vi "log analysis_gps.vi"() -> ()   [LabVIEW 2018] (continued)
,0.0976,0.1029,4.9518,0f000001,0*3a7eab6c\n\tsystem status\tnormal 2 27.800000 0 0\trobot status\t227.318577\t105.493966\t8.215100\t0.358371\t-1.600174\t171.393514\t0.252000\t0.087000\n\t\n15:37:15.7\tlog_raw\tgps_raw\t#INSPVAXA,USB3,0,48.5,FINESTEERING,2107,283053.700,02000000,471d,15824;INS_ALIGNMENT_COMPLETE,INS_RTKFIXED,37.37108102802,126.72339980538,8.2112,22.3000,0.0729,-0.2744,-0.0174,0.330552076,-1.494765101,278.139995916,0.4480,0.2956,0.5639,0.1143,0.0926,0.0779,0.0976,0.1029,4.9518,0f000001,0*6b892211\n\tsystem status\tnormal 2 27.800000 0 0\trobot status\t227.176950\t105.524570\t8.211200\t0.330552\t-1.494765\t171.860004\t0.412000\t-0.165000\n\t\n15:37:16.2\tlog_raw\tgps_raw\t#DUALANTENNAHEADINGA,USB3,0,45.5,FINESTEERING,2107,283054.200,02000000,d426,15824;INSUFFICIENT_OBS,NONE,-1.000000000,0.000000000,0.000000000,0.0,0.000000000,0.000000000,\"631T\",19,2,2,2,04,00,20,00*86f4b129\n\tsystem status\tnormal 2 27.800000 0 0\trobot status\t227.035841\t105.555084\t8.206800\t0.430368\t-1.501164\t172.299734\t0.195000\t0.158000\n\t\n15:37:16.7\tlog_raw\tgps_raw\t#INSPVAXA,USB3,0,45.5,FINESTEERING,2107,283054.700,02000000,471d,15824;INS_ALIGNMENT_COMPLETE,INS_RTKFIXED,37.37108154829,126.72339665209,8.2035,22.3000,0.0578,-0.2607,-0.0176,0.280593250,-1.428439620,277.446082188,0.4484,0.2957,0.5646,0.1144,0.0926,0.0779,0.0976,0.1029,4.9527,0f000001,0*8d0f64c8\n\tsystem status\tnormal 2 27.900000 0 0\trobot status\t226.897637\t105.582319\t8.203500\t0.280593\t-1.428440\t172.553918\t0.233000\t0.103000\n\t\n15:37:17.2\tlog_raw\tgps_raw\t#INSPVAXA,USB3,0,46.0,FINESTEERING,2107,283055.200,02000000,471d,15824;INS_ALIGNMENT_COMPLETE,INS_RTKFIXED,37.37108179458,126.72339508506,8.2008,22.3000,0.0590,-0.2687,-0.0093,0.251526173,-1.446507840,277.289322874,0.4481,0.2956,0.5644,0.1143,0.0926,0.0779,0.0976,0.1029,4.9538,0f000001,0*05040f15\n\tsystem status\tnormal 2 27.900000 0 0\trobot status\t226.758832\t105.609657\t8.200800\t0.251526\t-1.446508\t172.710677\t0.330000\t-0.056000\n\t\n15:37:17.7\tlog_raw\tgps_raw\t#INSPVAXA,USB3,0,46.0,FINESTEERING,2107,283055.700,02000000,471d,15824;INS_ALIGNMENT_COMPLETE,INS_RTKFIXED,37.37108204101,126.72339350294,8.1980,22.3000,0.0573,-0.2710,-0.0141,0.338881932,-1.408720439,277.315135363,0.4481,0.2956,0.5644,0.1143,0.0926,0.0779,0.0976,0.1029,4.9538,0f000001,0*6debbe04\n\tsystem status\tnormal 2 27.900000 0 0\trobot status\t226.618691\t105.637011\t8.198000\t0.338882\t-1.408720\t172.684865\t0.289000\t0.007000\n\t\n15:37:18.2\tlog_raw\tgps_raw\t#INSPVAXA,USB3,0,52.0,FINESTEERING,2107,283056.200,02000000,471d,15824;INS_ALIGNMENT_COMPLETE,INS_RTKFIXED,37.37108228588,126.72339196103,8.1952,22.3000,0.0487,-0.2508,-0.0076,0.405017158,-1.170976426,277.337977168,0.4477,0.2956,0.5639,0.1144,0.0926,0.0778,0.0976,0.1028,4.9548,0f000001,0*8b541580\n\tsystem status\tnormal 2 27.900000 0 0\trobot status\t226.482111\t105.664192\t8.195200\t0.405017\t-1.170976\t172.662023\t0.253000\t0.037000\n\t\n15:37:18.7\tlog_raw\tgps_raw\t#DUALANTENNAHEADINGA,USB3,0,52.0,FINESTEERING,2107,283056.700,02000000,d426,15824;INSUFFICIENT_OBS,NONE,-1.000000000,0.000000000,0.000000000,0.0,0.000000000,0.000000000,\"631T\",13,2,2,2,04,00,20,00*95485060\n\tsystem status\tnormal 2 28.000000 0 0\trobot status\t226.354812\t105.690997\t8.192600\t0.493668\t-1.115925\t172.765731\t0.208000\t0.011000\n\t\n15:37:19.2\tlog_raw\tgps_raw\t#DUALANTENNAHEADINGA,USB3,0,50.0,FINESTEERING,2107,283057.200,02000000,d426,15824;INSUFFICIENT_OBS,NONE,-1.000000000,0.000000000,0.000000000,0.0,0.000000000,0.000000000,\"631T\",13,2,2,2,04,00,20,00*e70ae8a8\n\tsystem status\tnormal 2 27.900000 0 0\trobot status\t226.254411\t105.711039\t8.190300\t0.338108\t-0.961096\t172.566593\t0.336000\t0.019000\n\t\n15:37:19.7\tlog_raw\tgps_raw\t#DUALANTENNAHEADINGA,USB3,0,50.0,FINESTEERING,2107,283057.700,02000000,d426,15824;INSUFFICIENT_OBS,NONE,-1.000000000,0.000000000,0.000000000,0.0,0.000000000,0.000000000,\"631T\",13,2,2,2,04,00,20,00*3019f9f1\n\tsystem status\tnormal 2 28.000000 0 0\trobot status\t226.091572\t105.739836\t8.186700\t0.308993\t-0.921996\t172.531902\t0.231000\t-0.008000\n\t\n15:37:20.2\tlog_raw\tgps_raw\t#INSPVAXA,USB3,0,52.0,FINESTEERING,2107,283058.200,02000000,471d,15824;INS_ALIGNMENT_COMPLETE,INS_RTKFIXED,37.37108315467,126.72338641713,8.1848,22.3000,0.0560,-0.2718,-0.0107,0.129590736,-0.819774204,277.698102716,0.4474,0.2955,0.5631,0.1155,0.0927,0.0778,0.0975,0.1028,4.9554,0f000001,0*a6d9a945\n\tsystem status\tnormal 2 27.900000 0 0\trobot status\t225.991041\t105.760627\t8.184800\t0.129591\t-0.819774\t172.301897\t0.296000\t-0.040000\n\t\n15:37:20.7\tlog_raw\tgps_raw\t#INSPVAXA,USB3,0,52.0,FINESTEERING,2107,283058.700,02000000,471d,15824;INS_ALIGNMENT_COMPLETE,INS_RTKFIXED,37.37108344441,126.72338455262,8.1832,22.3000,0.0621,-0.2653,-0.0184,0.032268015,-0.987434909,277.857905932,0.4474,0.2955,0.5631,0.1155,0.0927,0.0778,0.0975,0.1028,4.9554,0f000001,0*0fff6d0e\n\tsystem status\tnormal 2 28.000000 0 0\trobot status\t225.825886\t105.792788\t8.183200\t0.032268\t-0.987435\t172.142094\t0.338000\t0.019000\n\t\n15:37:21.2\tlog_raw\tgps_raw\t#INSPVAXA,USB3,0,51.0,FINESTEERING,2107,283059.200,02000000,471d,15824;INS_ALIGNMENT_COMPLETE,INS_RTKFIXED,37.37108373104,126.72338298116,8.1814,22.3000,0.0640,-0.2840,-0.0248,0.084962299,-0.861930897,278.528163453,0.4480,0.2954,0.5625,0.1142,0.0926,0.0777,0.0975,0.1027,4.9533,0f000001,0*55180826\n\tsystem status\tnormal 2 27.900000 0 0\trobot status\t225.686688\t105.824604\t8.181400\t0.084962\t-0.861931\t171.471837\t0.294000\t-0.065000\n\t\n15:37:21.7\tlog_raw\tgps_raw\t#INSPVAXA,USB3,0,51.0,FINESTEERING,2107,283059.700,02000000,471d,15824;INS_ALIGNMENT_COMPLETE,INS_RTKFIXED,37.37108405973,126.72338145683,8.1789,22.3000,0.0766,-0.2838,-0.0077,0.302314246,-0.745003967,279.694826311,0.4480,0.2954,0.5625,0.1142,0.0926,0.0777,0.0975,0.1027,4.9533,0f000001,0*c3a85521\n\tsystem status\tnormal 2 27.800000 0 0\trobot status\t225.551666\t105.861087\t8.178900\t0.302314\t-0.745004\t170.305174\t0.268000\t-0.122000\n\t\n15:37:22.2\tlog_raw\tgps_raw\t#DUALANTENNAHEADINGA,USB3,0,49.5,FINESTEERING,2107,283060.200,02000000,d426,15824;INSUFFICIENT_OBS,NONE,-1.000000000,0.000000000,0.000000000,0.0,0.000000000,0.000000000,\"631T\",14,2,2,2,04,00,20,00*d9be019d\n\tsystem status\tnormal 2 27.700000 0 0\trobot status\t225.411173\t105.899741\t8.176500\t0.188888\t-0.758738\t168.859131\t0.270000\t-0.100000\n\t\n15:37:22.7\tlog_raw\tgps_raw\t#INSPVAXA,USB3,0,49.5,FINESTEERING,2107,283060.700,02000000,471d,15824;INS_ALIGNMENT_COMPLETE,INS_RTKFIXED,37.37108477080,126.72337829109,8.1755,22.3000,0.0829,-0.2746,-0.0191,-0.114275154,-0.865621982,282.712324181,0.4478,0.2952,0.5620,0.1144,0.0926,0.0777,0.0975,0.1027,4.9522,0f000001,0*f5ce6e6a\n\tsystem status\tnormal 2 27.700000 0 0\trobot status\t225.271250\t105.940012\t8.175500\t-0.114275\t-0.865622\t167.287676\t0.300000\t-0.060000\n\t\n15:37:23.2\tlog_raw\tgps_raw\t#DUALANTENNAHEADINGA,USB3,0,49.0,FINESTEERING,2107,283061.200,02008000,d426,15824;SOL_COMPUTED,L1_FLOAT,-1.000000000,252.567794800,53.338584900,0.0,294.937744141,135.460769653,\"631T\",15,6,6,6,04,00,20,23*fbe42f58\n\tsystem status\tnormal 2 27.600000 0 0\trobot status\t225.132703\t105.985425\t8.176200\t-0.269945\t-1.010706\t165.810739\t0.300000\t-0.051000\n\t\n15:37:23.7\tlog_raw\tgps_raw\t#DUALANTENNAHEADINGA,USB3,0,49.0,FINESTEERING,2107,283061.700,02008000,d426,15824;INSUFFICIENT_OBS,NONE,-1.000000000,0.000000000,0.000000000,0.0,0.000000000,0.000000000,\"631T\",13,2,2,2,04,00,20,00*6aa2fd3b\n\tsystem status\tnormal 2 27.700000 0 0\trobot status\t224.997401\t106.035994\t8.177700\t-0.281716\t-0.789311\t164.588174\t0.297000\t-0.033000\n\t\n15:37:24.2\tlog_raw\tgps_raw\t#DUALANTENNAHEADINGA,USB3,0,45.5,FINESTEERING,2107,283062.200,02008000,d426,15824;INSUFFICIENT_OBS,NONE,-1.000000000,0.000000000,0.000000000,0.0,0.000000000,0.000000000,\"631T\",13,2,2,2,04,00,20,00*8005e2b6\n\tsystem status\tnormal 2 27.700000 0 0\trobot status\t224.859892\t106.090568\t8.178500\t-0.217716\t-0.817210\t163.548657\t0.247000\t-0.094000\n\t\n15:37:24.7\tlog_raw\tgps_raw\t#DUALANTENNAHEADINGA,USB3,0,45.5,FINESTEERING,2107,283062.700,02008000,d426,15824;INSUFFICIENT_OBS,NONE,-1.000000000,0.000000000,0.000000000,0.0,0.000000000,0.000000000,\"631T\",13,2,2,2,04,00,20,00*5716f3ef\n\tsystem status\tnormal 2 27.800000 0 0\trobot status\t224.725412\t106.145668\t8.178100\t-0.361245\t-0.626933\t162.778759\t0.341000\t0.060000\n\t\n15:37:25.2\tlog_raw\tgps_raw\t#DUALANTENNAHEADINGA,USB3,0,46.0,FINESTEERING,2107,283063.200,02008000,d426,15824;INSUFFICIENT_OBS,NONE,-1.000000000,0.000000000,0.000000000,0.0,0.000000000,0.000000000,\"631T\",12,2,2,2,04,00,20,00*c388fb17\n\tsystem status\tnormal 2 27.800000 0 0\trobot status\t224.590934\t106.202616\t8.177500\t-0.366610\t-0.485076\t162.261228\t0.254000\t-0.071000\n\t\n15:37:25.7\tlog_raw\tgps_raw\t#INSPVAXA,USB3,0,46.0,FINESTEERING,2107,283063.700,02008000,471d,15824;INS_ALIGNMENT_COMPLETE,INS_RTKFIXED,37.37108763910,126.72336915850,8.1772,22.3000,0.0613,-0.1484,-0.0057,-0.315544156,-0.705788351,288.188502375,0.4460,0.2952,0.5608,0.1140,0.0926,0.0776,0.0975,0.1026,4.9515,0f000001,0*11521a0a\n\tsystem status\tnormal 2 27.900000 0 0\trobot status\t224.462300\t106.258371\t8.177200\t-0.315544\t-0.705788\t161.811498\t0.183000\t-0.002000\n\t\n15:37:26.2\tlog_raw\tgps_raw\t#DUALANTENNAHEADINGA,USB3,0,49.5,FINESTEERING,2107,283064.200,02008000,d426,15824;INSUFFICIENT_OBS,NONE,-1.000000000,0.000000000,0.000000000,0.0,0.000000000,0.000000000,\"631T\",14,2,2,2,04,00,20,00*a33c9019\n\tsystem status\tnormal 2 28.000000 0 0\trobot status\t224.458512\t106.272057\t8.177700\t-0.418271\t-0.580192\t162.096787\t0.000000\t0.000000\n\t\n15:37:26.7\tlog_raw\tgps_raw\t#DUALANTENNAHEADINGA,USB3,0,49.5,FINESTEERING,2107,283064.700,02008000,d426,15824;INSUFFICIENT_OBS,NONE,-1.000000000,0.000000000,0.000000000,0.0,0.000000000,0.000000000,\"631T\",13,2,2,2,04,00,20,00*3e110a0b\n\tsystem status\tnormal 2 28.000000 0 0\trobot status\t224.462166\t106.283022\t8.179100\t-0.421246\t-0.578710\t162.036915\t0.000000\t0.000000\n\t\n15:37:27.2\tlog_raw\tgps_raw\t#DUALANTENNAHEADINGA,USB3,0,50.0,FINESTEERING,2107,283065.200,02008000,d426,15824;INSUFFICIENT_OBS,NONE,-1.000000000,0.000000000,0.000000000,0.0,0.000000000,0.000000000,\"631T\",13,2,2,2,04,00,20,00*f0ffb566\n\tsystem status\tnormal 2 28.000000 0 0\trobot status\t224.465375\t106.293143\t8.180100\t-0.419277\t-0.578107\t162.046332\t0.000000\t0.000000\n\t\n15:37:27.7\tlog_raw\tgps_raw\t#DUALANTENNAHEADINGA,USB3,0,50.0,FINESTEERING,2107,283065.700,02008000,d426,15824;INSUFFICIENT_OBS,NONE,-1.000000000,0.000000000,0.000000000,0.0,0.000000000,0.000000000,\"631T\",14,2,2,2,04,00,20,00*6dd22f74\n\tsystem status\tnormal 2 28.000000 0 0\trobot status\t224.467251\t106.301137\t8.180600\t-0.418596\t-0.575436\t162.044524\t0.000000\t0.000000\n\t\n15:37:28.2\tlog_raw\tgps_raw\t#DUALANTENNAHEADINGA,USB3,0,47.5,FINESTEERING,2107,283066.200,02000000,d426,15824;INSUFFICIENT_OBS,NONE,-1.000000000,0.000000000,0.000000000,0.0,0.000000000,0.000000000,\"631T\",15,2,2,2,04,00,20,00*afd2d569\n\tsystem status\tnormal 2 28.000000 0 0\trobot status\t224.469165\t106.307513\t8.181000\t-0.417828\t-0.575071\t162.040318\t0.000000\t0.000000\n\t\n15:37:28.7\tlog_raw\tgps_raw\t#INSPVAXA,USB3,0,47.5,FINESTEERING,2107,283066.700,02000000,471d,15824;INS_ALIGNMENT_COMPLETE,INS_RTKFIXED,37.37108811035,126.72336925303,8.1815,22.3000,0.0201,0.0148,-0.0079,-0.417962669,-0.573305874,287.968672901,0.4491,0.2953,0.5602,0.1160,0.0930,0.0776,0.0974,0.1026,4.9384,0f000001,0*010a2d8b\n\tsystem status\tnormal 2 28.000000 0 0\trobot status\t224.470673\t106.310672\t8.181500\t-0.417963\t-0.573306\t162.031327\t0.000000\t0.000000\n\t\n15:37:29.2\tlog_raw\tgps_raw\t#INSPVAXA,USB3,0,49.5,FINESTEERING,2107,283067.200,02000000,471d,15824;INS_ALIGNMENT_COMPLETE,INS_RTKFIXED,37.37108813168,126.72336927578,8.1822,22.3000,0.0181,0.0163,-0.0073,-0.419452547,-0.574416189,287.977918899,0.4495,0.2954,0.5600,0.1153,0.0929,0.0776,0.0974,0.1026,4.9275,0f000001,0*549c769b\n\tsystem status\tnormal 2 28.000000 0 0\trobot status\t224.472688\t106.313040\t8.182200\t-0.419453\t-0.574416\t162.022081\t0.000000\t0.000000\n\t\n15:37:29.7\tlog_raw\tgps_raw\t#DUALANTENNAHEADINGA,USB3,0,49.5,FINESTEERING,2107,283067.700,02000000,d426,15824;INSUFFICIENT_OBS,NONE,-1.000000000,0.000000000,0.000000000,0.0,0.000000000,0.000000000,\"631T\",12,2,2,2,04,00,20,00*49080399\n\tsystem status\tnormal 2 28.000000 0 0\trobot status\t224.474564\t106.313838\t8.183300\t-0.418041\t-0.575113\t162.011465\t0.000000\t0.000000\n\t\n15:37:30.2\tlog_raw\tgps_raw\t#DUALANTENNAHEADINGA,USB3,0,52.0,FINESTEERING,2107,283068.200,02000000,d426,15824;INSUFFICIENT_OBS,NONE,-1.000000000,0.000000000,0.000000000,0.0,0.000000000,0.000000000,\"631T\",10,2,2,2,04,00,20,00*54582190\n\tsystem status\tnormal 2 28.000000 0 0\trobot status\t224.476732\t106.314053\t8.184200\t-0.416762\t-0.574697\t162.002567\t0.000000\t0.000000\n\t\n15:37:30.7\tlog_raw\tgps_raw\t#DUALANTENNAHEADINGA,USB3,0,52.0,FINESTEERING,2107,283068.700,02000000,d426,15824;INSUFFICIENT_OBS,NONE,-1.000000000,0.000000000,0.000000000,0.0,0.000000000,0.000000000,\"631T\",10,2,2,2,04,00,20,00*834b30c9\n\tsystem status\tnormal 2 28.000000 0 0\trobot status\t224.477944\t106.313408\t8.184900\t-0.414613\t-0.574002\t161.993059\t0.000000\t0.000000\n\t\n15:37:31.2\tlog_raw\tgps_raw\t#DUALANTENNAHEADINGA,USB3,0,51.0,FINESTEERING,2107,283069.200,02000000,d426,15824;INSUFFICIENT_OBS,NONE,-1.000000000,0.000000000,0.000000000,0.0,0.000000000,0.000000000,\"631T\",10,2,2,2,04,00,20,00*954d5ea5\n\tsystem status\tnormal 2 28.000000 0 0\trobot status\t224.478944\t106.312623\t8.185800\t-0.413248\t-0.574345\t161.980835\t0.000000\t0.000000\n\t\n15:37:31.7\tlog_raw\tgps_raw\t#DUALANTENNAHEADINGA,USB3,0,51.0,FINESTEERING,2107,283069.700,02000000,d426,15824;INSUFFICIENT_OBS,NONE,-1.000000000,0.000000000,0.000000000,0.0,0.000000000,0.000000000,\"631T\",10,2,2,2,04,00,20,00*425e4ffc\n\tsystem status\tnormal 2 28.000000 0 0\trobot status\t224.478622\t106.311286\t8.187100\t-0.413743\t-0.575972\t161.971285\t0.000000\t0.000000\n\t\n15:37:32.2\tlog_raw\tgps_raw\t#DUALANTENNAHEADINGA,USB3,0,52.5,FINESTEERING,2107,283070.200,02000000,d426,15824;INSUFFICIENT_OBS,NONE,-1.000000000,0.000000000,0.000000000,0.0,0.000000000,0.000000000,\"631T\",10,2,2,2,04,00,20,00*26625f62\n\tsystem status\tnormal 2 28.000000 0 0\trobot status\t224.472931\t106.304441\t8.191500\t-0.413676\t-0.576142\t161.957409\t0.000000\t0.000000\n\t\n15:37:32.7\tlog_raw\tgps_raw\t#DUALANTENNAHEADINGA,USB3,0,52.5,FINESTEERING,2107,283070.700,02000000,d426,15824;INSUFFICIENT_OBS,NONE,-1.000000000,0.000000000,0.000000000,0.0,0.000000000,0.000000000,\"631T\",13,2,2,2,04,00,20,00*5227c892\n\tsystem status\tnormal 2 28.000000 0 0\trobot status\t224.457049\t106.286388\t8.201500\t-0.415988\t-0.580830\t161.940237\t0.000000\t0.000000\n\t\n15:37:33.2\tlog_raw\tgps_raw\t#DUALANTENNAHEADINGA,USB3,0,54.5,FINESTEERING,2107,283071.200,02000000,d426,15824;INSUFFICIENT_OBS,NONE,-1.000000000,0.000000000,0.000000000,0.0,0.000000000,0.000000000,\"631T\",13,2,2,2,04,00,20,00*6a072c8b\n\tsystem status\tnormal 2 28.000000 0 0\trobot status\t224.446581\t106.274894\t8.208600\t-0.417440\t-0.583830\t161.929639\t0.000000\t0.000000\n\t\n15:37:33.7\tlog_raw\tgps_raw\t\tsystem status\tnormal 2 28.000000 0 0\trobot status\t224.445080\t106.274741\t8.210500\t-0.413663\t-0.584668\t161.932180\t0.000000\t0.000000\n\t\n15:37:34.2\tlog_raw\tgps_raw\t#DUALANTENNAHEADINGA,USB3,0,49.5,FINESTEERING,2107,283072.200,02000000,d426,15824;INSUFFICIENT_OBS,NONE,-1.000000000,0.000000000,0.000000000,0.0,0.000000000,0.000000000,\"631T\",11,2,2,2,04,00,20,00*c3e637e1\n\tsystem status\tnormal 2 28.000000 0 0\trobot status\t224.444030\t106.274625\t8.212100\t-0.413003\t-0.586018\t161.934159\t0.000000\t0.000000\n\t\n15:37:34.7\tlog_raw\tgps_raw\t#DUALANTENNAHEADINGA,USB3,0,49.5,FINESTEERING,2107,283072.700,02000000,d426,15824;INSUFFICIENT_OBS,NONE,-1.000000000,0.000000000,0.000000000,0.0,0.000000000,0.000000000,\"631T\",13,2,2,2,04,00,20,00*60412049\n\tsystem status\tnormal 2 28.000000 0 0\trobot status\t224.443743\t106.274758\t8.213100\t-0.410619\t-0.587707\t161.938405\t0.000000\t0.000000\n\t\n15:37:35.2\tlog_raw\tgps_raw\t#DUALANTENNAHEADINGA,USB3,0,45.5,FINESTEERING,2107,283073.200,02000000,d426,15824;INSUFFICIENT_OBS,NONE,-1.000000000,0.000000000,0.000000000,0.0,0.000000000,0.000000000,\"631T\",13,2,2,2,04,00,20,00*042cd0ba\n\tsystem status\tnormal 2 28.000000 0 0\trobot status\t224.443799\t106.274913\t8.214000\t-0.409148\t-0.588494\t161.942929\t0.000000\t0.000000\n\t\n15:37:35.7\tlog_raw\tgps_raw\t#DUALANTENNAHEADINGA,USB3,0,45.5,FINESTEERING,2107,283073.700,02000000,d426,15824;INSUFFICIENT_OBS,NONE,-1.000000000,0.000000000,0.000000000,0.0,0.000000000,0.000000000,\"631T\",14,2,2,2,04,00,20,00*99014aa8\n\tsystem status\tnormal 2 28.000000 0 0\trobot status\t224.443802\t106.275172\t8.214400\t-0.408380\t-0.588614\t161.947579\t0.000000\t0.000000\n\t\n15:37:36.2\tlog_raw\tgps_raw\t#DUALANTENNAHEADINGA,USB3,0,50.0,FINESTEERING,2107,283074.200,02000000,d426,15824;INSUFFICIENT_OBS,NONE,-1.000000000,0.000000000,0.000000000,0.0,0.000000000,0.000000000,\"631T\",14,2,2,2,04,00,20,00*3ee80c21\n\tsystem status\tnormal 2 28.000000 0 0\trobot status\t224.443955\t106.275672\t8.214800\t-0.408998\t-0.591093\t161.953750\t0.000000\t0.000000\n\t\n15:37:36.7\tlog_raw\tgps_raw\t#DUALANTENNAHEADINGA,USB3,0,50.0,FINESTEERING,2107,283074.700,02000000,d426,15824;INSUFFICIENT_OBS,NONE,-1.000000000,0.000000000,0.000000000,0.0,0.000000000,0.000000000,\"631T\",13,2,2,2,04,00,20,00*a3c59633\n\tsystem status\tnormal 2 28.000000 0 0\trobot status\t224.443819\t106.276172\t8.215000\t-0.407165\t-0.589977\t161.958792\t0.000000\t0.000000\n\t\n15:37:37.2\tlog_raw\tgps_raw\t#DUALANTENNAHEADINGA,USB3,0,48.5,FINESTEERING,2107,283075.200,02000000,d426,15824;INSUFFICIENT_OBS,NONE,-1.000000000,0.000000000,0.000000000,0.0,0.000000000,0.000000000,\"631T\",14,2,2,2,04,00,20,00*435174b1\n\tsystem status\tnormal 2 28.000000 0 0\trobot status\t224.443749\t106.276912\t8.215400\t-0.406197\t-0.590364\t161.964407\t0.000000\t0.000000\n\t\n15:37:37.7\tlog_raw\tgps_raw\t#DUALANTENNAHEADINGA,USB3,0,48.5,FINESTEERING,2107,283075.700,02000000,d426,15824;INSUFFICIENT_OBS,NONE,-1.000000000,0.000000000,0.000000000,0.0,0.000000000,0.000000000,\"631T\",14,2,2,2,04,00,20,00*944265e8\n\tsystem status\tnormal 2 28.000000 0 0\trobot status\t224.444106\t106.277977\t8.215900\t-0.403240\t-0.589075\t161.971979\t0.000000\t0.000000\n\t\n15:37:38.2\tlog_raw\tgps_raw\t#DUALANTENNAHEADINGA,USB3,0,37.5,FINESTEERING,2107,283076.200,02000000,d426,15824;INSUFFICIENT_OBS,NONE,-1.000000000,0.000000000,0.000000000,0.0,0.000000000,0.000000000,\"631T\",12,2,2,2,04,00,20,00*42000f60\n\tsystem status\tnormal 2 28.000000 0 0\trobot status\t224.444412\t106.279441\t8.216500\t-0.402469\t-0.590649\t161.978968\t0.000000\t0.000000\n\t\n15:37:38.7\tlog_raw\tgps_raw\t#DUALANTENNAHEADINGA,USB3,0,37.5,FINESTEERING,2107,283076.700,02000000,d426,15824;INSUFFICIENT_OBS,NONE,-1.000000000,0.000000000,0.000000000,0.0,0.000000000,0.000000000,\"631T\",12,2,2,2,04,00,20,00*95131e39\n\tsystem status\tnormal 2 28.000000 0 0\trobot status\t224.444474\t106.280452\t8.217300\t-0.403001\t-0.589091\t161.987676\t0.000000\t0.000000\n\t\n15:37:39.2\tlog_raw\tgps_raw\t#DUALANTENNAHEADINGA,USB3,0,41.5,FINESTEERING,2107,283077.200,02000000,d426,15824;INSUFFICIENT_OBS,NONE,-1.000000000,0.000000000,0.000000000,0.0,0.000000000,0.000000000,\"631T\",13,2,2,2,04,00,20,00*225f994e\n\tsystem status\tnormal 2 28.000000 0 0\trobot status\t224.444454\t106.281759\t8.217900\t-0.403382\t-0.588903\t161.995009\t0.000000\t0.000000\n\t\n15:37:39.7\tlog_raw\tgps_raw\t#DUALANTENNAHEADINGA,USB3,0,41.5,FINESTEERING,2107,283077.700,02000000,d426,15824;INSUFFICIENT_OBS,NONE,-1.000000000,0.000000000,0.000000000,0.0,0.000000000,0.000000000,\"631T\",14,2,2,2,04,00,20,00*bf72035c\n\tsystem status\tnormal 2 28.000000 0 0\trobot status\t224.444326\t106.282784\t8.218400\t-0.402465\t-0.590017\t162.002959\t0.000000\t0.000000\n\t\n15:37:40.2\tlog_raw\tgps_raw\t\tsystem status\tnormal 2 28.000000 0 0\trobot status\t224.444423\t106.283924\t8.218700\t-0.402799\t-0.591657\t162.009798\t0.000000\t0.000000\n\t\n15:37:40.7\tlog_raw\tgps_raw\t#DUALANTENNAHEADINGA,USB3,0,47.5,FINESTEERING,2107,283078.700,02000000,d426,15824;INSUFFICIENT_OBS,NONE,-1.000000000,0.000000000,0.000000000,0.0,0.000000000,0.000000000,\"631T\",14,2,2,2,04,00,20,00*3fc2c0c1\n\tsystem status\tnormal 2 28.000000 0 0\trobot status\t224.444432\t106.284530\t8.218700\t-0.403496\t-0.590478\t162.017828\t0.000000\t0.000000\n\t\n15:37:41.2\tlog_raw\tgps_raw\t#INSPVAXA,USB3,0,47.0,FINESTEERING,2107,283079.250,02008000,471d,15824;INS_ALIGNMENT_COMPLETE,INS_RTKFIXED,37.37108788068,126.72336895793,8.2189,22.3000,0.0088,0.0013,-0.0012,-0.401485866,-0.591652619,287.973728649,0.2375,0.1652,0.3301,0.0344,0.0343,0.0312,0.0796,0.0806,4.8842,0f000005,0*b7c6e88e\n\tsystem status\tnormal 2 28.000000 0 0\trobot status\t224.444534\t106.285183\t8.218900\t-0.401486\t-0.591653\t162.026271\t0.000000\t0.000000\n\t\n15:37:41.7\tlog_raw\tgps_raw\t\tsystem status\tnormal 2 28.000000 0 0\trobot status\t224.445189\t106.285558\t8.219200\t-0.401801\t-0.589988\t162.030580\t0.000000\t0.000000\n\t\n15:37:42.2\tlog_raw\tgps_raw\t#DUALANTENNAHEADINGA,USB3,0,48.5,FINESTEERING,2107,283080.200,02008000,d426,15824;INSUFFICIENT_OBS,NONE,-1.000000000,0.000000000,0.000000000,0.0,0.000000000,0.000000000,\"631T\",14,2,2,2,04,00,20,00*53647ec7\n\tsystem status\tnormal 2 28.000000 0 0\trobot status\t224.445852\t106.286374\t8.219400\t-0.402906\t-0.589159\t162.034861\t0.000000\t0.000000\n\t\n15:37:42.7\tlog_raw\tgps_raw\t\tsystem status\tnormal 2 28.000000 0 0\trobot status\t224.446285\t106.286761\t8.219700\t-0.403955\t-0.586941\t162.040555\t0.000000\t0.000000\n\t\n15:37:43.2\tlog_raw\tgps_raw\t#DUALANTENNAHEADINGA,USB3,0,49.5,FINESTEERING,2107,283081.200,02008000,d426,15824;INSUFFICIENT_OBS,NONE,-1.000000000,0.000000000,0.000000000,0.0,0.000000000,0.000000000,\"631T\",13,2,2,2,04,00,20,00*10c627f1\n\tsystem status\tnormal 2 28.000000 0 0\trobot status\t224.446560\t106.287440\t8.219900\t-0.405217\t-0.586615\t162.044562\t0.000000\t0.000000\n\t\n15:37:43.7\tlog_raw\tgps_raw\t#DUALANTENNAHEADINGA,USB3,0,49.5,FINESTEERING,2107,283081.700,02008000,d426,15824;INSUFFICIENT_OBS,NONE,-1.000000000,0.000000000,0.000000000,0.0,0.000000000,0.000000000,\"631T\",13,2,2,2,04,00,20,00*c7d536a8\n\tsystem status\tnormal 2 28.000000 0 0\trobot status\t224.446108\t106.287608\t8.220600\t-0.406769\t-0.585328\t162.047588\t0.000000\t0.000000\n\t\n15:37:44.2\tlog_raw\tgps_raw\t#INSPVAXA,USB3,0,48.0,FINESTEERING,2107,283082.250,02008000,471d,15824;INS_ALIGNMENT_COMPLETE,INS_RTKFIXED,37.37108790543,126.72336897434,8.2212,22.3000,0.0087,0.0020,-0.0010,-0.406487889,-0.586741608,287.950772341,0.2277,0.1614,0.3135,0.0344,0.0343,0.0312,0.0796,0.0806,4.8871,0f000005,0*4c1cc0b2\n\tsystem status\tnormal 2 28.000000 0 0\trobot status\t224.445987\t106.287930\t8.221200\t-0.406488\t-0.586742\t162.049228\t0.000000\t0.000000\n\t\n15:37:44.7\tlog_raw\tgps_raw\t#DUALANTENNAHEADINGA,USB3,0,48.0,FINESTEERING,2107,283082.700,02008000,d426,15824;INSUFFICIENT_OBS,NONE,-1.000000000,0.000000000,0.000000000,0.0,0.000000000,0.000000000,\"631T\",13,2,2,2,04,00,20,00*40830bab\n\tsystem status\tnormal 2 28.000000 0 0\trobot status\t224.446132\t106.288223\t8.221600\t-0.406755\t-0.585861\t162.050623\t0.000000\t0.000000\n\t\n15:37:45.2\tlog_raw\tgps_raw\t#DUALANTENNAHEADINGA,USB3,0,51.0,FINESTEERING,2107,283083.200,02008000,d426,15824;INSUFFICIENT_OBS,NONE,-1.000000000,0.000000000,0.000000000,0.0,0.000000000,0.000000000,\"631T\",13,2,2,2,04,00,20,00*db17520a\n\tsystem status\tnormal 2 28.000000 0 0\trobot status\t224.446264\t106.288675\t8.222000\t-0.407177\t-0.586377\t162.052509\t0.000000\t0.000000\n\t\n15:37:45.7\tlog_raw\tgps_raw\t#INSPVAXA,USB3,0,51.0,FINESTEERING,2107,283083.750,02008000,471d,15824;INS_ALIGNMENT_COMPLETE,INS_RTKFIXED,37.37108791341,126.72336897923,8.2220,22.3000,0.0085,0.0022,-0.0015,-0.407747547,-0.586428741,287.947615621,0.2254,0.1606,0.3090,0.0344,0.0343,0.0312,0.0797,0.0806,4.8884,0f000005,0*f8c3e66c\n\tsystem status\tnormal 2 28.000000 0 0\trobot status\t224.446420\t106.288816\t8.222000\t-0.407748\t-0.586429\t162.052384\t0.000000\t0.000000\n\t\n15:37:46.2\tlog_raw\tgps_raw\t#DUALANTENNAHEADINGA,USB3,0,45.5,FINESTEERING,2107,283084.200,02008000,d426,15824;INSUFFICIENT_OBS,NONE,-1.000000000,0.000000000,0.000000000,0.0,0.000000000,0.000000000,\"631T\",11,2,2,2,04,00,20,00*bb1dd58f\n\tsystem status\tnormal 2 28.000000 0 0\trobot status\t224.446500\t106.289064\t8.222000\t-0.409198\t-0.586376\t162.053952\t0.000000\t0.000000\n\t\n15:37:46.7\tlog_raw\tgps_raw\t\tsystem status\tnormal 2 28.000000 0 0\trobot status\t224.446684\t106.288909\t8.222000\t-0.409062\t-0.587638\t162.053958\t0.000000\t0.000000\n\t\n15:37:47.2\tlog_raw\tgps_raw\t\tsystem status\tnormal 2 28.000000 0 0\trobot status\t224.446760\t106.288952\t8.221800\t-0.410007\t-0.586377\t162.057124\t0.000000\t0.000000\n\t\n15:37:47.7\tlog_raw\tgps_raw\t#DUALANTENNAHEADINGA,USB3,0,52.0,FINESTEERING,2107,283085.700,02008000,d426,15824;INSUFFICIENT_OBS,NONE,-1.000000000,0.000000000,0.000000000,0.0,0.000000000,0.000000000,\"631T\",13,2,2,2,04,00,20,00*17682428\n\tsystem status\tnormal 2 28.000000 0 0\trobot status\t224.446389\t106.288861\t8.222200\t-0.411301\t-0.588650\t162.058541\t0.000000\t0.000000\n\t\n15:37:48.2\tlog_raw\tgps_raw\t#DUALANTENNAHEADINGA,USB3,0,48.5,FINESTEERING,2107,283086.200,02008000,d426,15824;INSUFFICIENT_OBS,NONE,-1.000000000,0.000000000,0.000000000,0.0,0.000000000,0.000000000,\"631T\",11,2,2,2,04,00,20,00*da4fefea\n\tsystem status\tnormal 2 28.000000 0 0\trobot status\t224.446063\t106.289003\t8.222700\t-0.413828\t-0.587587\t162.058759\t0.000000\t0.000000\n\t\n15:37:48.7\tlog_raw\tgps_raw\t#INSPVAXA,USB3,0,48.5,FINESTEERING,2107,283086.750,02008000,471d,15824;INS_ALIGNMENT_COMPLETE,INS_RTKFIXED,37.37108790964,126.72336897431,8.2231,22.3000,0.0055,-0.0003,-0.0011,-0.414418876,-0.584788673,287.941437407,0.2201,0.1591,0.2978,0.0344,0.0343,0.0312,0.0796,0.0806,4.8926,0f000005,0*39edc872\n\tsystem status\tnormal 2 28.000000 0 0\trobot status\t224.445985\t106.288397\t8.223100\t-0.414419\t-0.584789\t162.058563\t0.000000\t0.000000\n\t\n15:37:49.2\tlog_raw\tgps_raw\t#INSPVAXA,USB3,0,50.0,FINESTEERING,2107,283087.250,02000000,471d,15824;INS_ALIGNMENT_COMPLETE,INS_RTKFIXED,37.37108790633,126.72336897138,8.2235,22.3000,0.0050,-0.0003,-0.0013,-0.412674863,-0.583241565,287.941135781,0.2189,0.1588,0.2948,0.0344,0.0343,0.0312,0.0796,0.0806,4.8941,0f000005,0*d8c4a8b8\n\tsystem status\tnormal 2 28.000000 0 0\trobot status\t224.445725\t106.288030\t8.223500\t-0.412675\t-0.583242\t162.058864\t0.000000\t0.000000\n\t\n15:37:49.7\tlog_raw\tgps_raw\t#INSPVAXA,USB3,0,50.0,FINESTEERING,2107,283087.750,02000000,471d,15824;INS_ALIGNMENT_COMPLETE,INS_RTKFIXED,37.37108790910,126.72336896298,8.2239,22.3000,0.0060,-0.0018,-0.0010,-0.411196763,-0.583056579,287.939929568,0.2189,0.1588,0.2948,0.0344,0.0343,0.0312,0.0796,0.0806,4.8941,0f000005,0*cc42fb84\n\tsystem status\tnormal 2 28.000000 0 0\trobot status\t224.444981\t106.288337\t8.223900\t-0.411197\t-0.583057\t162.060070\t0.000000\t0.000000\n\t\n15:37:50.2\tlog_raw\tgps_raw\t\tsystem status\tnormal 2 28.000000 0 0\trobot status\t224.444527\t106.288674\t8.224200\t-0.409646\t-0.581615\t162.061103\t0.000000\t0.000000\n\t\n15:37:50.7\tlog_raw\tgps_raw\t#INSPVAXA,USB3,0,51.5,FINESTEERING,2107,283088.750,02000000,471d,15824;INS_ALIGNMENT_COMPLETE,INS_RTKFIXED,37.37108791273,126.72336896374,8.2243,22.3000,0.0059,-0.0008,-0.0019,-0.408020685,-0.578100141,287.936827542,0.2178,0.1585,0.2920,0.0344,0.0343,0.0312,0.0796,0.0806,4.8955,0f000005,0*8a62d2d3\n\tsystem status\tnormal 2 28.000000 0 0\trobot status\t224.445048\t106.288740\t8.224300\t-0.408021\t-0.578100\t162.063172\t0.000000\t0.000000\n\t\n15:37:51.2\tlog_raw\tgps_raw\t#DUALANTENNAHEADINGA,USB3,0,50.5,FINESTEERING,2107,283089.200,02000000,d426,15824;INSUFFICIENT_OBS,NONE,-1.000000000,0.000000000,0.000000000,0.0,0.000000000,0.000000000,\"631T\",11,2,2,2,04,00,20,00*8b9cc3ca\n\tsystem status\tnormal 2 28.000000 0 0\trobot status\t224.445401\t106.288825\t8.224500\t-0.406223\t-0.580268\t162.064808\t0.000000\t0.000000\n\t\n15:37:51.7\tlog_raw\tgps_raw\t#DUALANTENNAHEADINGA,USB3,0,50.5,FINESTEERING,2107,283089.700,02000000,d426,15824;INSUFFICIENT_OBS,NONE,-1.000000000,0.000000000,0.000000000,0.0,0.000000000,0.000000000,\"631T\",12,2,2,2,04,00,20,00*ffd9543a\n\tsystem status\tnormal 2 28.000000 0 0\trobot status\t224.445480\t106.288658\t8.224900\t-0.404941\t-0.578839\t162.065780\t0.000000\t0.000000\n\t\n15:37:52.2\tlog_raw\tgps_raw\t#INSPVAXA,USB3,0,48.0,FINESTEERING,2107,283090.250,02000000,471d,15824;INS_ALIGNMENT_COMPLETE,INS_RTKFIXED,37.37108791260,126.72336897396,8.2253,22.3000,0.0056,0.0014,-0.0008,-0.404918336,-0.579813079,287.934409966,0.2159,0.1581,0.2871,0.0344,0.0343,0.0312,0.0796,0.0806,4.8985,0f000005,0*237dfef6\n\tsystem status\tnormal 2 28.000000 0 0\trobot status\t224.445954\t106.288726\t8.225300\t-0.404918\t-0.579813\t162.065590\t0.000000\t0.000000\n\t\n15:37:52.7\tlog_raw\tgps_raw\t#INSPVAXA,USB3,0,48.0,FINESTEERING,2107,283090.750,02000000,471d,15824;INS_ALIGNMENT_COMPLETE,INS_RTKFIXED,37.37108791340,126.72336897831,8.2257,22.3000,0.0060,0.0017,-0.0005,-0.406200324,-0.580436127,287.932734672,0.2159,0.1581,0.2871,0.0344,0.0343,0.0312,0.0796,0.0806,4.8985,0f000005,0*2244ce35\n\tsystem status\tnormal 2 28.000000 0 0\trobot status\t224.446339\t106.288815\t8.225700\t-0.406200\t-0.580436\t162.067265\t0.000000\t0.000000\n\t\n15:37:53.2\tlog_raw\tgps_raw\t#DUALANTENNAHEADINGA,USB3,0,52.0,FINESTEERING,2107,283091.200,02000000,d426,15824;INSUFFICIENT_OBS,NONE,-1.000000000,0.000000000,0.000000000,0.0,0.000000000,0.000000000,\"631T\",10,2,2,2,04,00,20,00*e6cd9028\n\tsystem status\tnormal 2 28.000000 0 0\trobot status\t224.446582\t106.288910\t8.225900\t-0.405950\t-0.578270\t162.068375\t0.000000\t0.000000\n\t\n15:37:53.7\tlog_raw\tgps_raw\t#INSPVAXA,USB3,0,52.0,FINESTEERING,2107,283091.750,02000000,471d,15824;INS_ALIGNMENT_COMPLETE,INS_RTKFIXED,37.37108791121,126.72336898157,8.2259,22.3000,0.0063,0.0022,-0.0001,-0.406191825,-0.576334644,287.931619498,0.2151,0.1580,0.2849,0.0344,0.0343,0.0312,0.0796,0.0806,4.9000,0f000005,0*09e92407\n\tsystem status\tnormal 2 28.000000 0 0\trobot status\t224.446628\t106.288572\t8.225900\t-0.406192\t-0.576335\t162.068381\t0.000000\t0.000000\n\t\n15:37:54.2\tlog_raw\tgps_raw\t#DUALANTENNAHEADINGA,USB3,0,46.5,FINESTEERING,2107,283092.200,02008000,d426,15824;INSUFFICIENT_OBS,NONE,-1.000000000,0.000000000,0.000000000,0.0,0.000000000,0.000000000,\"631T\",12,2,2,2,04,00,20,00*fc458629\n\tsystem status\tnormal 2 28.000000 0 0\trobot status\t224.446924\t106.288587\t8.226000\t-0.405917\t-0.575151\t162.068129\t0.000000\t0.000000\n\t\n15:37:54.7\tlog_raw\tgps_raw\t#INSPVAXA,USB3,0,46.5,FINESTEERING,2107,283092.750,02008000,471d,15824;INS_ALIGNMENT_COMPLETE,INS_RTKFIXED,37.37108790953,126.72336899162,8.2261,22.3000,0.0061,0.0038,0.0006,-0.405842887,-0.574777504,287.928097277,0.2145,0.1579,0.2830,0.0344,0.0343,0.0312,0.0796,0.0806,4.9014,0f000005,0*3b1b2e95\n\tsystem status\tnormal 2 28.000000 0 0\trobot status\t224.447518\t106.288385\t8.226100\t-0.405843\t-0.574778\t162.071903\t0.000000\t0.000000\n\t\n15:37:55.2\tlog_raw\tgps_raw\t#DUALANTENNAHEADINGA,USB3,0,46.5,FINESTEERING,2107,283093.200,02008000,d426,15824;INSUFFICIENT_OBS,NONE,-1.000000000,0.000000000,0.000000000,0.0,0.000000000,0.000000000,\"631T\",12,2,2,2,04,00,20,00*919d82f0\n\tsystem status\tnormal 2 28.000000 0 0\trobot status\t224.448060\t106.288233\t8.226200\t-0.407052\t-0.576383\t162.073166\t0.000000\t0.000000\n\t\n15:37:55.7\tlog_raw\tgps_raw\t#INSPVAXA,USB3,0,46.5,FINESTEERING,2107,283093.750,02008000,471d,15824;INS_ALIGNMENT_COMPLETE,INS_RTKFIXED,37.37108790514,126.72336900394,8.2261,22.3000,0.0049,0.0045,0.0000,-0.407478337,-0.576861946,287.929394509,0.2139,0.1578,0.2812,0.0344,0.0343,0.0312,0.0796,0.0806,4.9028,0f000005,0*f255cd77\n\tsystem status\tnormal 2 28.000000 0 0\trobot status\t224.448609\t106.287898\t8.226100\t-0.407478\t-0.576862\t162.070605\t0.000000\t0.000000\n\t\n15:37:56.2\tlog_raw\tgps_raw\t#INSPVAXA,USB3,0,49.5,FINESTEERING,2107,283094.250,02008000,471d,15824;INS_ALIGNMENT_COMPLETE,INS_RTKFIXED,37.37108790174,126.72336900960,8.2259,22.3000,0.0041,0.0045,-0.0005,-0.407655175,-0.578418030,287.928618080,0.2134,0.1577,0.2795,0.0344,0.0343,0.0312,0.0796,0.0805,4.9042,0f000005,0*67a4f1a6\n\tsystem status\tnormal 2 28.000000 0 0\trobot status\t224.449111\t106.287520\t8.225900\t-0.407655\t-0.578418\t162.071382\t0.000000\t0.000000\n\t\n15:37:56.7\tlog_raw\tgps_raw\t#INSPVAXA,USB3,0,49.5,FINESTEERING,2107,283094.750,02008000,471d,15824;INS_ALIGNMENT_COMPLETE,INS_RTKFIXED,37.37108789686,126.72336901475,8.2257,22.3000,0.0044,0.0046,-0.0012,-0.406458944,-0.580608983,287.928943902,0.2134,0.1577,0.2795,0.0344,0.0343,0.0312,0.0796,0.0805,4.9042,0f000005,0*f975bb71\n\tsystem status\tnormal 2 28.000000 0 0\trobot status\t224.449567\t106.286979\t8.225700\t-0.406459\t-0.580609\t162.071056\t0.000000\t0.000000\n\t\n15:37:57.2\tlog_raw\tgps_raw\t#DUALANTENNAHEADINGA,USB3,0,46.0,FINESTEERING,2107,283095.200,02008000,d426,15824;INSUFFICIENT_OBS,NONE,-1.000000000,0.000000000,0.000000000,0.0,0.000000000,0.000000000,\"631T\",15,2,2,2,04,00,20,00*3978f3e0\n\tsystem status\tnormal 2 28.000000 0 0\trobot status\t224.449966\t106.286906\t8.225600\t-0.406369\t-0.580278\t162.070846\t0.000000\t0.000000\n\t\n15:37:57.7\tlog_raw\tgps_raw\t#INSPVAXA,USB3,0,46.0,FINESTEERING,2107,283095.750,02008000,471d,15824;INS_ALIGNMENT_COMPLETE,INS_RTKFIXED,37.37108789802,126.72336901889,8.2258,22.3000,0.0057,0.0037,-0.0015,-0.407856141,-0.581296268,287.930403916,0.2130,0.1576,0.2780,0.0344,0.0343,0.0312,0.0795,0.0805,4.9056,0f000005,0*89459e2d\n\tsystem status\tnormal 2 28.000000 0 0\trobot status\t224.449933\t106.287108\t8.225800\t-0.407856\t-0.581296\t162.069596\t0.000000\t0.000000\n\t\n15:37:58.2\tlog_raw\tgps_raw\t#INSPVAXA,USB3,0,44.5,FINESTEERING,2107,283096.250,02000000,471d,15824;INS_ALIGNMENT_COMPLETE,INS_RTKFIXED,37.37108790052,126.72336901738,8.2259,22.3000,0.0066,0.0026,-0.0012,-0.409158540,-0.581176612,287.930571782,0.2126,0.1576,0.2766,0.0344,0.0343,0.0312,0.0795,0.0805,4.9071,0f000005,0*d38b9ae0\n\tsystem status\tnormal 2 28.000000 0 0\trobot status\t224.449800\t106.287385\t8.225900\t-0.409159\t-0.581177\t162.069428\t0.000000\t0.000000\n\t\n15:37:58.7\tlog_raw\tgps_raw\t#INSPVAXA,USB3,0,44.5,FINESTEERING,2107,283096.750,02000000,471d,15824;INS_ALIGNMENT_COMPLETE,INS_RTKFIXED,37.37108790177,126.72336901650,8.2263,22.3000,0.0066,0.0025,-0.0011,-0.409708018,-0.580992332,287.931343125,0.2126,0.1576,0.2766,0.0344,0.0343,0.0312,0.0795,0.0805,4.9071,0f000005,0*11cd3564\n\tsystem status\tnormal 2 28.000000 0 0\trobot status\t224.449722\t106.287524\t8.226300\t-0.409708\t-0.580992\t162.068657\t0.000000\t0.000000\n\t\n15:37:59.2\tlog_raw\tgps_raw\t#INSPVAXA,USB3,0,50.0,FINESTEERING,2107,283097.250,02000000,471d,15824;INS_ALIGNMENT_COMPLETE,INS_RTKFIXED,37.37108790174,126.72336901580,8.2265,22.3000,0.0063,0.0024,-0.0010,-0.411930313,-0.582541736,287.929452176,0.2123,0.1575,0.2753,0.0344,0.0343,0.0312,0.0795,0.0805,4.9086,0f000005,0*85d40b4e\n\tsystem status\tnormal 2 28.000000 0 0\trobot status\t224.449660\t106.287520\t8.226500\t-0.411930\t-0.582542\t162.070548\t0.000000\t0.000000\n\t\n15:37:59.7\tlog_raw\tgps_raw\t#INSPVAXA,USB3,0,50.0,FINESTEERING,2107,283097.750,02000000,471d,15824;INS_ALIGNMENT_COMPLETE,INS_RTKFIXED,37.37108790027,126.72336901488,8.2267,22.3000,0.0062,0.0022,-0.0007,-0.412766504,-0.583030959,287.927282231,0.2123,0.1575,0.2753,0.0344,0.0343,0.0312,0.0795,0.0805,4.9086,0f000005,0*89dff8ff\n\tsystem status\tnormal 2 28.000000 0 0\trobot status\t224.449578\t106.287357\t8.226700\t-0.412767\t-0.583031\t162.072718\t0.000000\t0.000000\n\t\n15:38:00.2\tlog_raw\tgps_raw\t#INSPVAXA,USB3,0,48.5,FINESTEERING,2107,283098.250,02000000,471d,15824;INS_ALIGNMENT_COMPLETE,INS_RTKFIXED,37.37108790003,126.72336901347,8.2268,22.3000,0.0066,0.0014,-0.0006,-0.413922974,-0.582701162,287.926560126,0.2120,0.1575,0.2742,0.0344,0.0343,0.0312,0.0795,0.0805,4.9101,0f000005,0*70ee257d\n\tsystem status\tnormal 2 28.000000 0 0\trobot status\t224.449453\t106.287331\t8.226800\t-0.413923\t-0.582701\t162.073440\t0.000000\t0.000000\n\t\n15:38:00.7\tlog_raw\tgps_raw\t#INSPVAXA,USB3,0,48.5,FINESTEERING,2107,283098.750,02000000,471d,15824;INS_ALIGNMENT_COMPLETE,INS_RTKFIXED,37.37108789759,126.72336901204,8.2269,22.3000,0.0059,0.0011,-0.0001,-0.414260974,-0.583807411,287.925600594,0.2120,0.1575,0.2742,0.0344,0.0343,0.0312,0.0795,0.0805,4.9101,0f000005,0*03dc57a5\n\tsystem status\tnormal 2 28.000000 0 0\trobot status\t224.449327\t106.287060\t8.226900\t-0.414261\t-0.583807\t162.074399\t0.000000\t0.000000\n\t\n15:38:01.2\tlog_raw\tgps_raw\t#INSPVAXA,USB3,0,49.0,FINESTEERING,2107,283099.250,02000000,471d,15824;INS_ALIGNMENT_COMPLETE,INS_RTKFIXED,37.37108789570,126.72336901200,8.2271,22.3000,0.0061,0.0012,0.0001,-0.415797201,-0.582658490,287.926983863,0.2118,0.1575,0.2731,0.0344,0.0343,0.0312,0.0795,0.0805,4.9116,0f000005,0*b658d869\n\tsystem status\tnormal 2 28.000000 0 0\trobot status\t224.449323\t106.286850\t8.227100\t-0.415797\t-0.582658\t162.073016\t0.000000\t0.000000\n\t\n15:38:01.7\tlog_raw\tgps_raw\t\tsystem status\tnormal 2 28.000000 0 0\trobot status\t224.449613\t106.286708\t8.227100\t-0.415716\t-0.583247\t162.074731\t0.000000\t0.000000\n\t\n15:38:02.2\tlog_raw\tgps_raw\t#INSPVAXA,USB3,0,51.5,FINESTEERING,2107,283100.250,02000000,471d,15824;INS_ALIGNMENT_COMPLETE,INS_RTKFIXED,37.37108789328,126.72336901997,8.2271,22.3000,0.0052,0.0025,0.0001,-0.415319706,-0.581468435,287.925172452,0.2115,0.1574,0.2721,0.0344,0.0343,0.0312,0.0795,0.0805,4.9131,0f000005,0*eafa8938\n\tsystem status\tnormal 2 28.000000 0 0\trobot status\t224.450029\t106.286582\t8.227100\t-0.415320\t-0.581468\t162.074828\t0.000000\t0.000000\n\t\n15:38:02.7\tlog_raw\tgps_raw\t\tsystem status\tnormal 2 28.000000 0 0\trobot status\t224.450431\t106.286077\t8.226900\t-0.416162\t-0.580128\t162.076775\t0.000000\t0.000000\n\t\n15:38:03.2\tlog_raw\tgps_raw\t#INSPVAXA,USB3,0,51.5,FINESTEERING,2107,283101.250,02000000,471d,15824;INS_ALIGNMENT_COMPLETE,INS_RTKFIXED,37.37108788280,126.72336902694,8.2267,22.3000,0.0032,0.0031,0.0001,-0.415895315,-0.578950026,287.923664941,0.2113,0.1574,0.2712,0.0344,0.0343,0.0312,0.0795,0.0805,4.9145,0f000005,0*44540dbc\n\tsystem status\tnormal 2 28.000000 0 0\trobot status\t224.450647\t106.285418\t8.226700\t-0.415895\t-0.578950\t162.076335\t0.000000\t0.000000\n\t\n15:38:03.7\tlog_raw\tgps_raw\t#INSPVAXA,USB3,0,51.5,FINESTEERING,2107,283101.750,02000000,471d,15824;INS_ALIGNMENT_COMPLETE,INS_RTKFIXED,37.37108787688,126.72336902839,8.2270,22.3000,0.0029,0.0036,0.0002,-0.417826855,-0.580147759,287.923061019,0.2113,0.1574,0.2712,0.0344,0.0343,0.0312,0.0795,0.0805,4.9145,0f000005,0*aaec6ebb\n\tsystem status\tnormal 2 28.000000 0 0\trobot status\t224.450775\t106.284761\t8.227000\t-0.417827\t-0.580148\t162.076939\t0.000000\t0.000000\n\t\n15:38:04.2\tlog_raw\tgps_raw\t#INSPVAXA,USB3,0,47.0,FINESTEERING,2107,283102.250,02000000,471d,15824;INS_ALIGNMENT_COMPLETE,INS_RTKFIXED,37.37108787301,126.72336903085,8.2270,22.3000,0.0026,0.0034,0.0000,-0.417491423,-0.580282079,287.923862604,0.2111,0.1574,0.2703,0.0344,0.0343,0.0312,0.0795,0.0805,4.9158,0f000005,0*ceb9045c\n\tsystem status\tnormal 2 28.000000 0 0\trobot status\t224.450993\t106.284332\t8.227000\t-0.417491\t-0.580282\t162.076137\t0.000000\t0.000000\n\t\n15:38:04.7\tlog_raw\tgps_raw\t#INSPVAXA,USB3,0,47.0,FINESTEERING,2107,283102.750,02000000,471d,15824;INS_ALIGNMENT_COMPLETE,INS_RTKFIXED,37.37108787295,126.72336903129,8.2268,22.3000,0.0030,0.0034,0.0005,-0.416932840,-0.582279475,287.924574839,0.2111,0.1574,0.2703,0.0344,0.0343,0.0312,0.0795,0.0805,4.9158,0f000005,0*3c34a6bf\n\tsystem status\tnormal 
